vi "CRYGraph Step Socket.vi"(9 "sData":string, 10 "Queue Name":string, 11 "sAction":string) -> (3 "sDataOut":string)   [LabVIEW 2013]
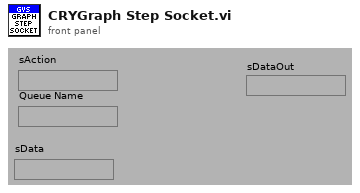
[diagram p1: front panel]
types:
  T1 = typedef "Graph Main Info Cluster.ctl" = cluster{"Selected_BarIdx":i32, "Selected_PanelIdx":i32, "Graph Main VIRef":refnum<vi>, "ToolBarClick":bool, "Spliter Ref Array":refnum<vi>[], "Panel Ref Array":refnum<vi>[], "Spliter_matrix":i32[][], "Panel_matrix":i32[][], "child_spliterIdx_matrix":i32[][], "split_pos_matrix":i32[][], "Title State":bool, "sQueueName":string, "Frame nID":i32, "Graph VIRef Array":cluster{"Graph VIRef":refnum<vi>, "Panel Idx":i32, "Frame VIRef":refnum<vi>, "Icon Ring":i32, "Graph Type":string}[], "View Type":string}
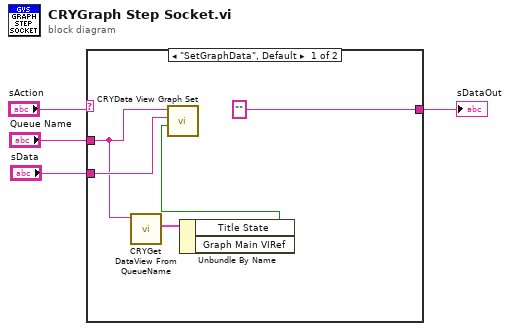
[diagram p0: block diagram]
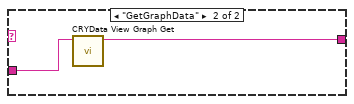
[diagram p2: hidden frame]
diagram:
  n1 = case shown="\"SetGraphData\", Default" "sAction" {
    tunnel: ["" ("Flattened Graph Property") w11] -> w2
    tunnel: "sData" -> [w8 _]
    tunnel: "Queue Name" -> [w7 w10]
    frame "SetGraphData", Default {
      n2 = call "CRYGet DataView From QueueName.vi"("DataView QueueName"=w7) -> ("DataView out"=w6:T1)  [unwired: 8 in, 2 out]
      n3 = Unbundle By Name(w6) -> ("Title State"=w5:bool)  [unwired: 1 out]
      n4 = call "CRYData View Graph Set.vi"("Title State"=w5, "Flattened Graph ViewPro"=w8, "Queue Name"=w7) -> ()  [unwired: 9 in]
    }
    frame "GetGraphData" {
      n5 = call "CRYData View Graph Get.vi"("Queue Name"=w10) -> ("Flattened Graph ViewPro"=w11:string)  [unwired: 10 in]
    }
  }
  "sDataOut" <- w2
